vi "FileIO-Experiment VIs Path.vi"(4 "relpath":string) -> (1 "full path":path)   [LabVIEW 2020]
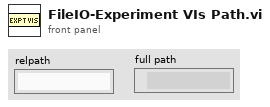
[diagram p1: front panel]
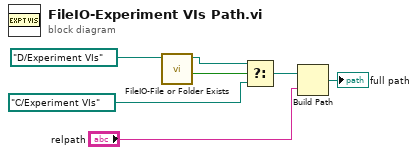
[diagram p0: block diagram]
diagram:
  n1 = call "FileIO-File or Folder Exists.vi"("path"=path "D:/Experiment VIs") -> ("Exists?"=w6:bool, "dup path"=w5:path)  [unwired: 7 in, 2 out]
  n2 = Select(t=w5, s=w6, f=path "C:/Experiment VIs") -> (s? t:f=w3:path)
  n3 = Build Path(base path=w3, name or relative path="relpath") -> (appended path=→"full path":path)
